vi "GetControlConstructor.vi"(7 "PythonConverter_GUI in":refnum<class "PythonConverter_GUI.lvclass">, 8 "error in":errorcluster, 11 "Control in":refnum<class "Control.lvclass">) -> (0 "error out":errorcluster, 1 "class":string, 2 "get image":bool, 3 "Control out":refnum<class "Control.lvclass">, 4 "module":T1, 5 "PythonConverter_GUI out":refnum<class "PythonConverter_GUI.lvclass">, 6 "constructor":string)   [LabVIEW 2014, in "PythonConverter_GUI.lvclass"]
uses:
  PythonConverter_GUI.lvclass
  VI Interpreter/Classes/Control/Control.lvclass
  TypeDefs/PythonModuleTD.ctl
  VI Interpreter/Classes/Control/Control.lvclass/Control.ctl
  VI Interpreter/Classes/Numeric/Numeric.lvclass
  VI Interpreter/Classes/Knob/Knob.lvclass
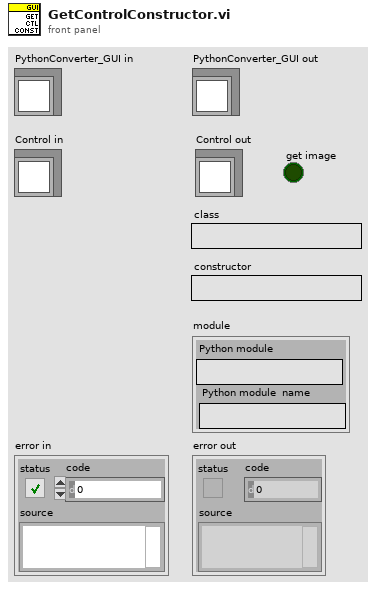
[diagram p1: front panel]
types:
  T1 = typedef "PythonConverter_GUI.lvclass/PythonModuleTD.ctl" = cluster{"Python module":string, "Python module  name":string}
  T2 = typedef "PythonConverter_GUI.lvclass/ConstructorInfo.ctl" = cluster{"Style ID":u32, "python class":string, "python module":string, "python module name":string, "check datatype":bool, "get image":bool}
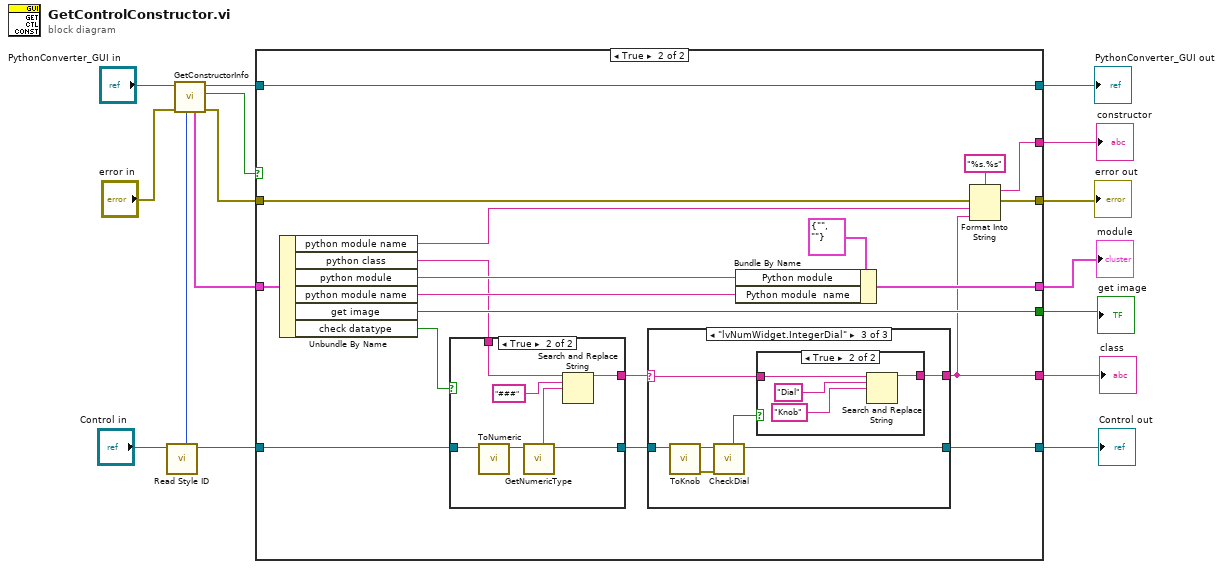
[diagram p0: block diagram]
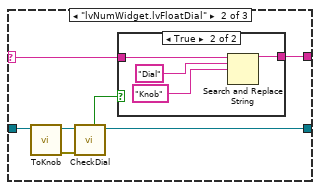
[diagram p4: hidden frame]
diagram:
  n1 = call "Read Style ID.vi"("Control in"="Control in") -> ("Control out"=w5:refnum<class "Control.lvclass">, "Style ID"=w14:u32)  [unwired: 7 in]
  n2 = call "GetConstructorInfo.vi"("Style ID"=w14, "error in"="error in", "PythonConverter_GUI in"="PythonConverter_GUI in") -> ("error out"=w9:errorcluster, "found"=w13:bool, "PythonConverter_GUI out"=w12:refnum<class "PythonConverter_GUI.lvclass">, "Constructor Info"=w10:T2)  [unwired: 5 in]
  n3 = case shown="True" w13 {
    tunnel: w12 -> [w18 w37]
    tunnel: w10 -> [_ w38]
    tunnel: w9 -> [w19 w34]
    tunnel: [w18 w37] -> w8
    tunnel: [w19 w33] -> w7
    tunnel: [w17 w23] -> w6
    tunnel: w5 -> [w17 w26]
    tunnel: [_ w29] -> w4
    tunnel: [_ w28] -> w3
    tunnel: [_ w21] -> w2
    tunnel: [_ w20] -> w1
    frame False {
    }
    frame True {
      n4 = Unbundle By Name(w38) -> ("python module name"=w36:string, "python class"=w22:string, "python module"=w31:string, "python module name"=w30:string, "get image"=w28:bool, "check datatype"=w27:bool)
      n5 = case shown="True" w27 {
        tunnel: w26 -> [w66 w73]
        tunnel: [w66 w71] -> w24
        tunnel: w22 -> [w65 w70]
        tunnel: [w65 w67] -> w25
        frame False {
        }
        frame True {
          n6 = call "ToNumeric.vi"("Generic"=w73) -> ("Numeric out"=w72:refnum<class "Numeric.lvclass">)  [unwired: 9 in, 1 out]
          n7 = call "GetNumericType.vi"("Numeric in"=w72) -> ("Numeric out"=w71:refnum<class "Numeric.lvclass">, "String"=w68:string)  [unwired: 6 in, 1 out]
          n8 = Search and Replace String(input string=w70, search string="###", replace string=w68) -> (result string=w67:string)  [unwired: 5 in, 3 out]
        }
      }
      n9 = case shown="\"lvNumWidget.IntegerDial\"" w25 {
        selector: w25 -> [w40 w42 w54]
        tunnel: w24 -> [w39 w47 w59]
        tunnel: [w39 w43 w55] -> w23
        tunnel: [w40 w41 w53] -> w21
        frame Default {
        }
        frame "lvNumWidget.lvFloatDial" {
          n10 = call "ToKnob.vi"("Generic"=w47) -> ("error out"=w45:errorcluster, "Knob out"=w46:refnum<class "Knob.lvclass">)  [unwired: 9 in]
          n11 = call "CheckDial.vi"("error in"=w45, "Knob in"=w46) -> ("Knob out"=w43:refnum<class "Knob.lvclass">, "Knob"=w44:bool)  [unwired: 4 in, 2 out]
          n12 = case shown="True" w44 {
            tunnel: w42 -> [w48 w52]
            tunnel: [w48 w49] -> w41
            frame False {
            }
            frame True {
              n13 = Search and Replace String(input string=w52, search string="Dial", replace string="Knob" ("replace string (\"\")")) -> (result string=w49:string)  [unwired: 5 in, 3 out]
            }
          }
        }
        frame "lvNumWidget.IntegerDial" {
          n14 = call "ToKnob.vi"("Generic"=w59) -> ("error out"=w57:errorcluster, "Knob out"=w58:refnum<class "Knob.lvclass">)  [unwired: 9 in]
          n15 = call "CheckDial.vi"("error in"=w57, "Knob in"=w58) -> ("Knob out"=w55:refnum<class "Knob.lvclass">, "Knob"=w56:bool)  [unwired: 4 in, 2 out]
          n16 = case shown="True" w56 {
            tunnel: w54 -> [w60 w64]
            tunnel: [w60 w61] -> w53
            frame False {
            }
            frame True {
              n17 = Search and Replace String(input string=w64, search string="Dial", replace string="Knob" ("replace string (\"\")")) -> (result string=w61:string)  [unwired: 5 in, 3 out]
            }
          }
        }
      }
      n18 = Bundle By Name(cluster=T1 {"Python module"="", "Python module  name"=""} ("module"), "Python module"=w31, "Python module  name"=w30) -> (w29:T1)
      n19 = Format Into String(format string="%s.%s", error in=w34, w36, w21) -> (resulting string=w20:string, error out=w33:errorcluster)  [unwired: 1 in]
    }
  }
  "error out" <- w7
  "Control out" <- w6
  "class" <- w2
  "module" <- w4
  "PythonConverter_GUI out" <- w8
  "get image" <- w3
  "constructor" <- w1
